vi "Reserve Sessions.vi"   [LabVIEW 2020, in "MeasurementLink Measurement Server.lvlib" / "Measure Call Context.lvclass"]
doc: "Reserves session(s) based on the provided pin information."
uses:
  Measure Call Context.lvclass
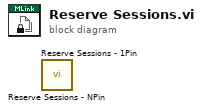
[diagram p0: block diagram]
diagram:
  n1 = call "Reserve Sessions - NPin.vi"() -> ()  [unwired: 9 in, 3 out]
  n2 = call "Reserve Sessions - 1Pin.vi"() -> ()  [unwired: 9 in, 3 out]
